vi "Write Text Frame.vi"(8 "error in (no error)":errorcluster, 9 "timeout (2000 ms)":i32=2000, 10 "Text":string, 11 "WebsocketsConnection in":refnum<class "WebsocketsConnection.lvclass">) -> (0 "error out":errorcluster, 3 "WebsocketsConnection out":refnum<class "WebsocketsConnection.lvclass">)   [LabVIEW 2013, in "MQTT_Websockets.lvlib" / "WebsocketsConnection.lvclass"]
doc: "This method shold not be used in the context of MQTT over Websockets.\nIt is being included in the library to allow for testing requirement MQTT-6.0.0-1 which specifies that an entity receiveing anything other than a binary frame should close the connection immediately."
uses:
  WebsocketsConnection.lvclass
  WebsocketsConnection.lvclass/WebsocketsConnection.ctl
  <vilib>/MediaMongrels Ltd/WebSockets/WebSockets/WebSocket/WebSocket.lvclass
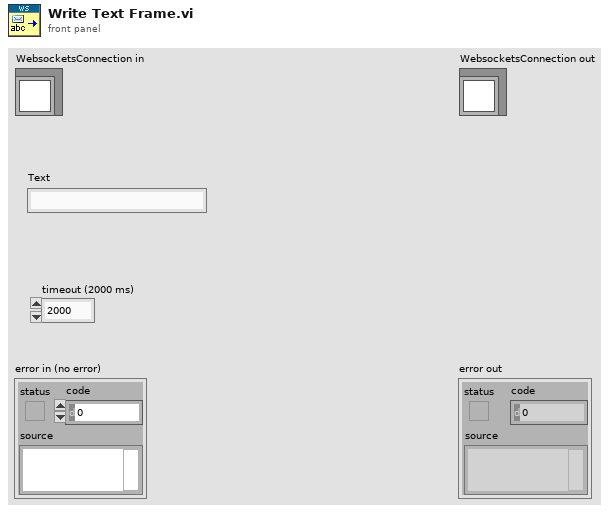
[diagram p1: front panel]
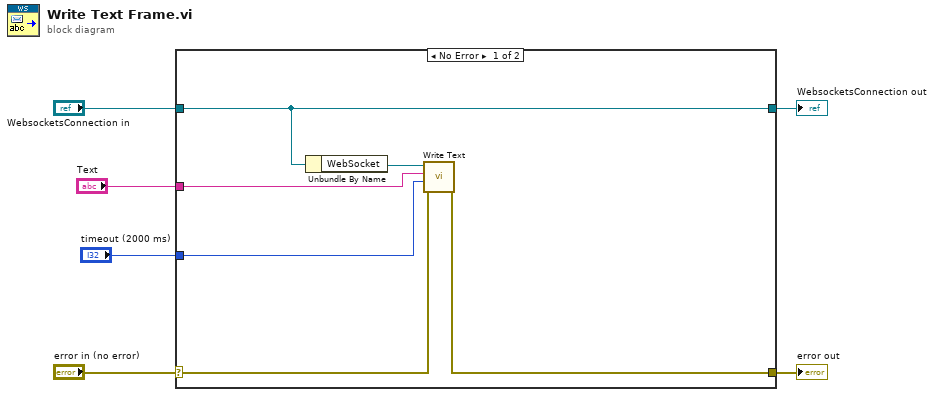
[diagram p0: block diagram]
diagram:
  n1 = case shown="No Error" "error in (no error)" {
    selector: "error in (no error)" -> [w8 w14]
    tunnel: [w7 w14] -> w5
    tunnel: [w12 w13] -> w3
    tunnel: "WebsocketsConnection in" -> [w12 w13]
    tunnel: "Text" -> [w10 _]
    tunnel: "timeout (2000 ms)" -> [w9 _]
    frame No Error {
      n2 = Unbundle By Name(w12) -> ("WebSocket"=w11:refnum<class "WebSocket.lvclass">)
      n3 = call-dynamic "Write Text.vi"("error in (no error)"=w8, "timeout ms (5000)"=w9, "String Data"=w10, "WebSocket in"=w11) -> ("error out"=w7:errorcluster)  [unwired: 6 in, 1 out]
    }
    frame Error {
    }
  }
  "error out" <- w5
  "WebsocketsConnection out" <- w3
